vi "PID_Caller.vi"() -> ()   [LabVIEW 2012]
panel:
  out "Waveform Chart":cluster{"Slide":dbl, "output":dbl}(graph)
  in  "stop":bool
  in  "output range":cluster{"output high":dbl, "output low":dbl}={"output high"=100.0, "output low"=-100.0}
  in  "PID gains":T1={"proportional gain (Kc)"=0.8, "integral time (Ti, min)"=0.0001, "derivative time (Td, min)"=1e-05} {"derivative time (Td, min)" format="%.5f"; "integral time (Ti, min)" format="%.5f"; "proportional gain (Kc)" format="%.5f"}
  in  "Slide":dbl(slide)=28.792569659442734 scale=-100.0..100.0
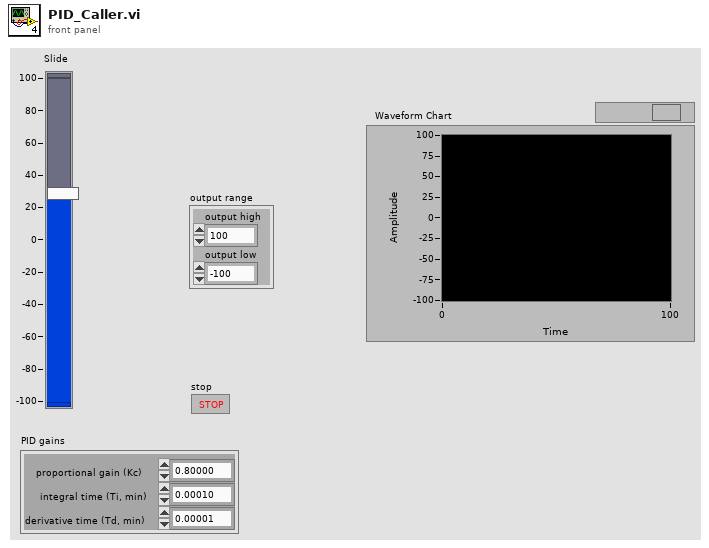
[diagram p1: front panel]
types:
  T1 = cluster{"proportional gain (Kc)":dbl, "integral time (Ti, min)":dbl, "derivative time (Td, min)":dbl}
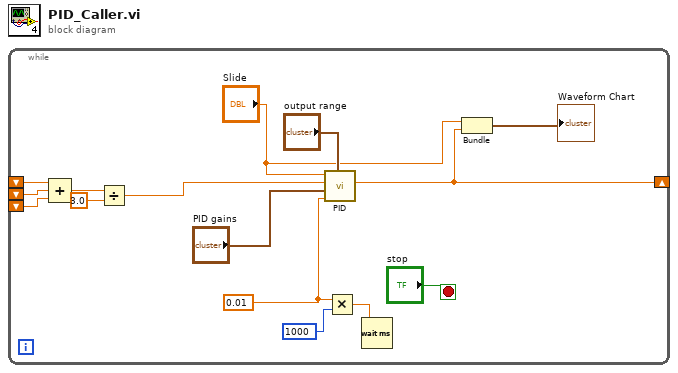
[diagram p0: block diagram]
diagram:
  n1 = while {
    shift-right: [w8] -> _
    shift-left: _ -> [w6]
    shift-left: _ -> [w5]
    shift-left: _ -> [w4]
    stop <- "stop" stop-if-true
    w11 = 0.01
    n2 = Compound Arithmetic op=ADD(w6, w5, w4) -> (w3:dbl)
    n3 = Divide(x=w3, y=3.0) -> (x/y=w2:dbl)
    n4 = call "PID.vi"("output range"="output range", "dt (s)"=w11, "PID gains"="PID gains", "process variable"=w2, "setpoint"="Slide") -> ("output"=w8:dbl)  [unwired: 6 in]
    n5 = Multiply(x=w11, y=1000) -> (x*y=w12:dbl)
    n6 = Wait (ms)(milliseconds to wait=w12) -> ()  [unwired: 1 out]
    n7 = Bundle("Slide"="Slide", "output"=w8) -> (→"Waveform Chart":cluster{"Slide":dbl, "output":dbl})  [unwired: 1 in]
  }
